vi "ep_Y to D convert (Waveform).vi"(8 "error in (no error)":errorcluster, 11 "phase voltage waveforms":waveform(dbl)[](array[waveform])) -> (0 "error out":errorcluster, 3 "line voltage waveforms":waveform(dbl)[](array[waveform]))   [LabVIEW 2014, in "NI_EP_Power Quality.lvlib"]
uses:
  <vilib>/addons/Electrical Power/PQ/NI_EP_Power Quality.lvlib
  <vilib>/addons/Electrical Power/PQ/Common/Controls/ep_AI Data Channel.ctl
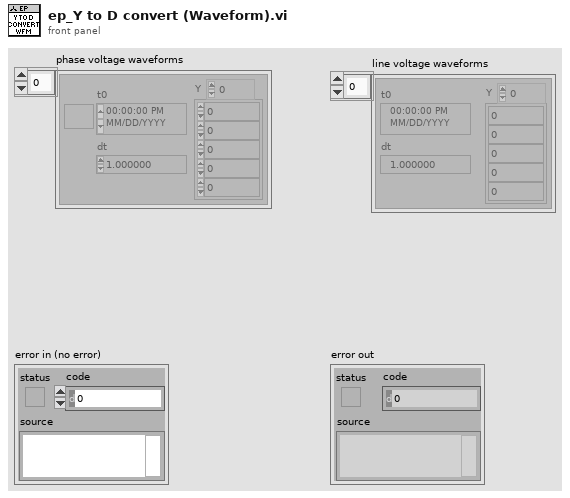
[diagram p1: front panel]
types:
  T1 = typedef "NI_EP_Power Quality.lvlib/ep_AI Data Channel.ctl" = enum16{"Voltage Phase A (L1)", "Voltage Phase B (L2)", "Voltage Phase C (L3)", "Voltage Phase N (Neutral)", "Current Phase A (L1)", "Current Phase B (L2)", "Current Phase C (L3)", "Current Phase N (Neutral)"}
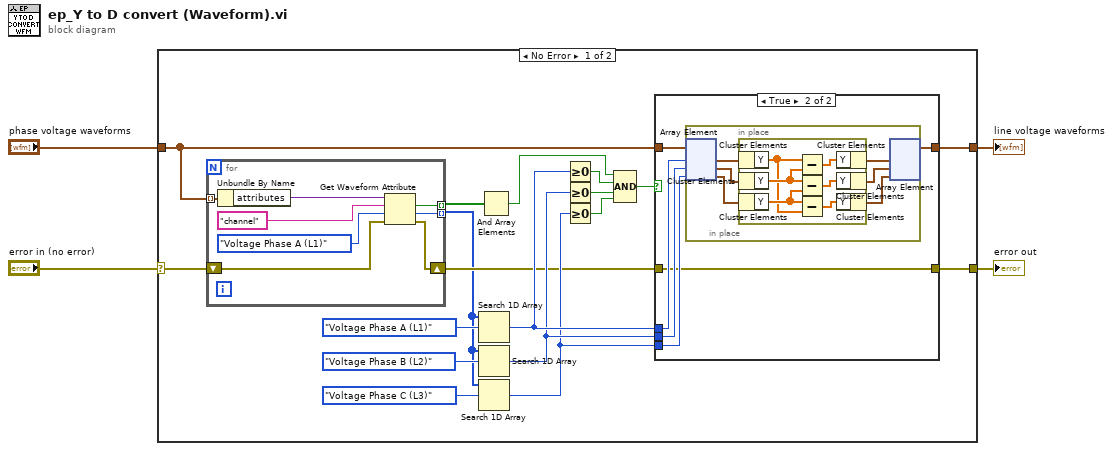
[diagram p0: block diagram]
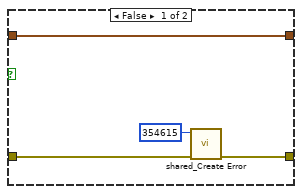
[diagram p2: hidden frame]
diagram:
  n1 = case shown="No Error" "error in (no error)" {
    selector: "error in (no error)" -> [w6 w53]
    tunnel: [w11 _] -> w4
    tunnel: "phase voltage waveforms" -> [w9 _]
    tunnel: [w7 w53] -> w2
    frame No Error {
      n2 = for {
        shift-right: [w26] -> w8
        shift-left: w6 -> [w27]
        tunnel: [w25] -> w10 mode=indexing
        tunnel: [w24] -> w5 mode=indexing
        tunnel: w9 -> [w23] mode=indexing
        n3 = Unbundle By Name(w23) -> ("attributes"=w28:variant)
        n4 = Get Waveform Attribute(4:w27, 5:ep_AI_Data_Channel."Voltage Phase A (L1)" ("AI data channel"), 6:"channel" ("name"), 7:w28) -> (0:w26:errorcluster, 1:w24:T1, 2:w25:bool)  [unwired: 1 out]
      }
      n5 = Search 1D Array(1D array=w5, element=ep_AI_Data_Channel."Voltage Phase A (L1)" ("AI data channel")) -> (index of element=w14:i32)  [unwired: 1 in]
      n6 = Search 1D Array(1D array=w5, element=ep_AI_Data_Channel."Voltage Phase B (L2)" ("AI data channel")) -> (index of element=w13:i32)  [unwired: 1 in]
      n7 = Search 1D Array(1D array=w5, element=ep_AI_Data_Channel."Voltage Phase C (L3)" ("AI data channel")) -> (index of element=w12:i32)  [unwired: 1 in]
      n8 = And Array Elements(Boolean array=w10) -> (logical AND=w16:bool)
      n9 = Greater Or Equal To 0?(x=w14) -> (x >= 0?=w17:bool)
      n10 = Greater Or Equal To 0?(x=w13) -> (x >= 0?=w21:bool)
      n11 = Greater Or Equal To 0?(x=w12) -> (x >= 0?=w22:bool)
      n12 = Compound Arithmetic op=AND(w16, w17, w21, w22) -> (w15:bool)
      n13 = case shown="True" w15 {
        tunnel: [w34 w36] -> w11
        tunnel: w9 -> [w34 w40]
        tunnel: w14 -> [_ w39]
        tunnel: w13 -> [_ w38]
        tunnel: w12 -> [_ w37]
        tunnel: w8 -> [w33 w35]
        tunnel: [w32 w35] -> w7
        frame False {
          n14 = call <vilib>:"shared_Create Error.vi"("error in (no error)"=w33, "error code (0)"=354615) -> ("error out"=w32:errorcluster)  [unwired: 9 in]
        }
        frame True {
          n15 = in-place {
            n16 = in-place-array #1(w40, w39, w38, w37) -> (w46:waveform(dbl), w45:waveform(dbl), w44:waveform(dbl))
            n17 = in-place {
              n18 = in-place-cluster #2(w46) -> ("Y"=w50:dbl[])
              n19 = in-place-cluster #3(w45) -> ("Y"=w52:dbl[])
              n20 = in-place-cluster #4(w44) -> ("Y"=w51:dbl[])
              n21 = Subtract(x=w50, y=w52) -> (x-y=w47:dbl[])
              n22 = Subtract(x=w52, y=w51) -> (x-y=w48:dbl[])
              n23 = Subtract(x=w51, y=w50) -> (x-y=w49:dbl[])
              n24 = in-place-cluster #2("Y"=w47) -> (w43:waveform(dbl))
              n25 = in-place-cluster #3("Y"=w48) -> (w42:waveform(dbl))
              n26 = in-place-cluster #4("Y"=w49) -> (w41:waveform(dbl))
            }
            n27 = in-place-array #1(w43, w42, w41) -> (w36:waveform(dbl)[])  [unwired: 3 out]
          }
        }
      }
    }
    frame Error {
    }
  }
  "error out" <- w2
  "line voltage waveforms" <- w4
